vi "rad_Get AppImage Properties.vi"(0 "AppImage Path":path=path "C:/dev/Architectures/Reference Designs/Application Deployment and Replication/Application Deployment Utility/trunk/source/Application Images/Blink.lvappimg", 5 "App Image Temp Folder":path, 7 "Show FP":bool, 11 "error in (no error)":errorcluster) -> (4 "Supported":bool, 6 "Current":bool, 8 "Older":bool, 10 "Newer":bool, 13 "AppImage Path":path=path "C:/dev/Architectures/Reference Designs/Application Deployment and Replication/Application Deployment Utility/trunk/source/Application Images/Blink.lvappimg", 14 "AppImage Properties":T1, 15 "error out":errorcluster)   [LabVIEW 2016]
uses:
  TypeDefs/rad_Application Image Properties.ctl
  TypeDefs/rad_FPGA Properties.ctl
  TypeDefs/rad_FPGA Flash Properties.ctl
  Util/FP Control/FP Control Functions.ctl
panel:
  # "Loading Application Image Properties ..."
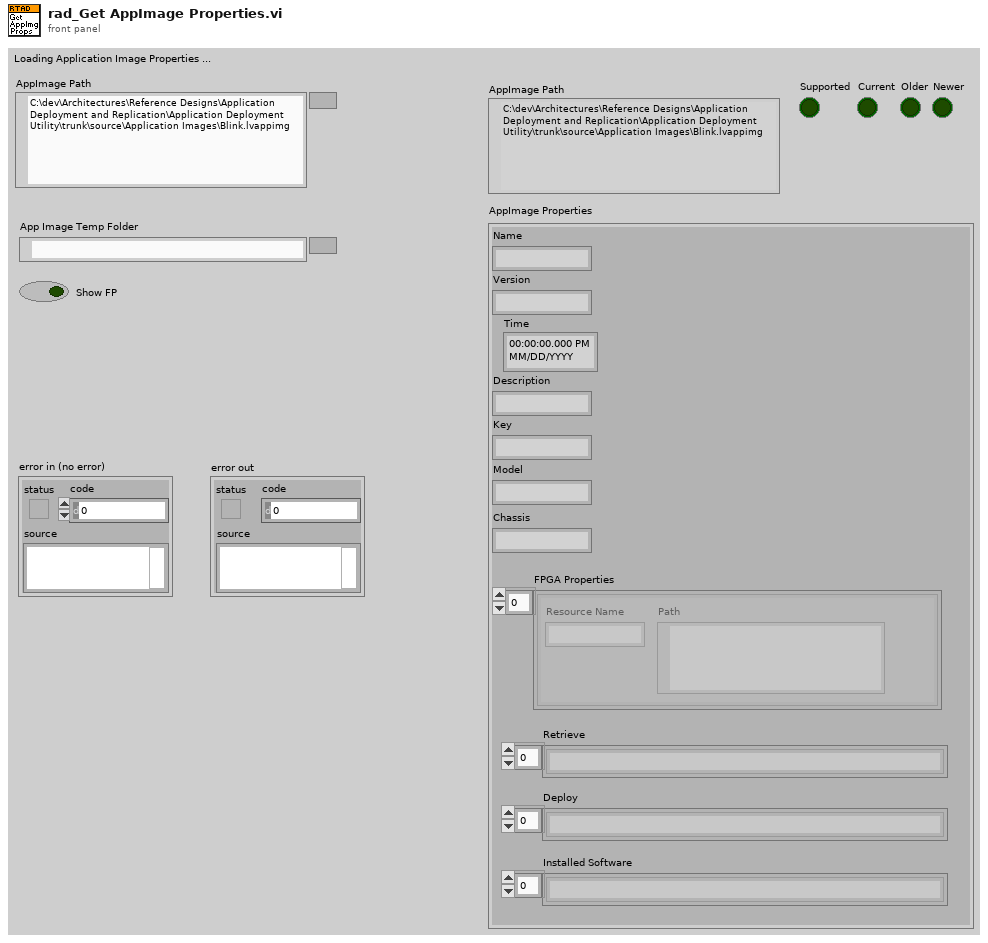
[diagram p1: front panel]
types:
  T1 = typedef "rad_Application Image Properties.ctl" = cluster{"Name":string, "Version":string, "Time":timestamp, "Description":string, "Key":string, "Chassis":string, "FPGA Properties":T2, "Model":string, "Retrieve":string[], "Deploy":string[], "Installed Software":string[]}
  T2 = typedef "rad_FPGA Properties.ctl" = T3[]
  T3 = typedef "rad_FPGA Flash Properties.ctl" = cluster{"Resource Name":string, "Path":path}
  T4 = typedef "FP Control Functions.ctl" = enum16{"Open", "Close", "Bring To Front", "Center"}
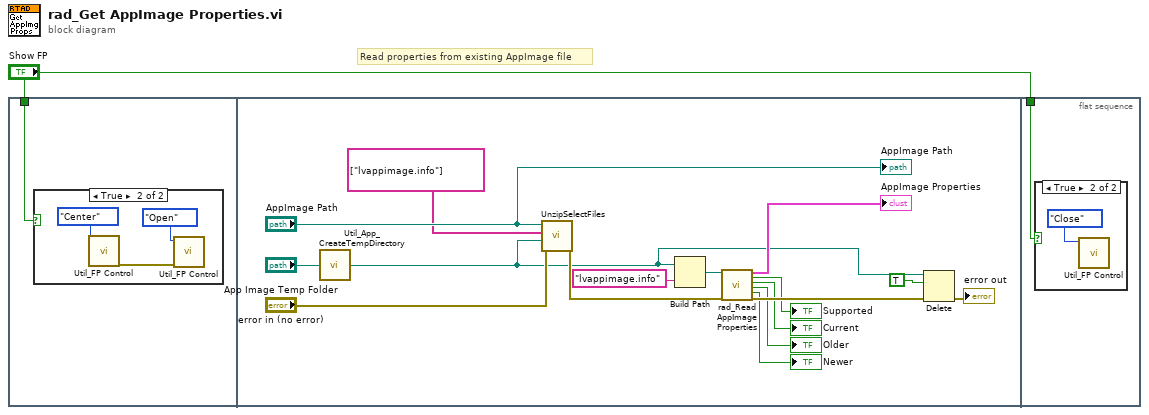
[diagram p0: block diagram]
diagram:
  # "Read properties from existing AppImage file"
  n1 = flat-sequence {
    tunnel: "Show FP" -> [w2]
    tunnel: "Show FP" -> [w22]
    frame #0 {
      n2 = case shown="True" w2 {
        frame False {
        }
        frame True {
          n3 = call "Util_FP Control.vi"("Function"=FP_Control_Functions."Center") -> ("error out"=w3:errorcluster)  [unwired: 1 in, 9 out]
          n4 = call "Util_FP Control.vi"("error in (no error)"=w3, "Function"=FP_Control_Functions."Open") -> ()  [unwired: 10 out]
        }
      }
    }
    frame #1 {
      n5 = call "Util_App_CreateTempDirectory.vi"("TempFolderPath"="App Image Temp Folder") -> ("TempFolderPath_out"=w6:path)
      n6 = call "UnzipSelectFiles.vi"("error in (no error)"="error in (no error)", "Target directory (same as Zip file if empty)"=w6, "Files to Unzip"=string[] ["lvappimage.info"], "Zip file"="AppImage Path") -> ("error out"=w15:errorcluster)  [unwired: 1 in, 6 out]
      n7 = Build Path(base path=w6, name or relative path="lvappimage.info") -> (appended path=w21:path)
      n8 = call "rad_Read AppImage Properties.vi"("AppImage Properties Path"=w21, "error in (no error)"=w15) -> ("AppImage Properties"=→"AppImage Properties":T1, "Supported"=→"Supported":bool, "Current"=→"Current":bool, "Older"=→"Older":bool, "Newer"=→"Newer":bool, "error out"=w12:errorcluster)  [unwired: 12 in]
      n9 = Delete(path (use dialog)=w6, entire hierarchy (F)=TRUE, error in=w12) -> (error out=→"error out":errorcluster)  [unwired: 4 out]
      "AppImage Path" <- "AppImage Path"
    }
    frame #2 {
      n10 = case shown="True" w22 {
        frame False {
        }
        frame True {
          n11 = call "Util_FP Control.vi"("Function"=FP_Control_Functions."Close") -> ()  [unwired: 1 in, 10 out]
        }
      }
    }
  }
